vi "GetPrinterSettings.vi"(8 "error in (no error)":errorcluster, 11 "PrintDialog Refnum":refnum<k24>) -> (0 "error out":errorcluster, 2 "printer settings":T1, 3 "Refnum Out":refnum<k24>)   [LabVIEW 2015]
uses:
  System.Windows.Forms
  System.Drawing
panel:
  in  "margins (1.00)":T2={"top"=1.0, "left"=1.0, "right"=1.0, "bottom"=1.0} {"right" format="%.2f"; "bottom" format="%.2f"; "top" format="%.2f"; "left" format="%.2f"}
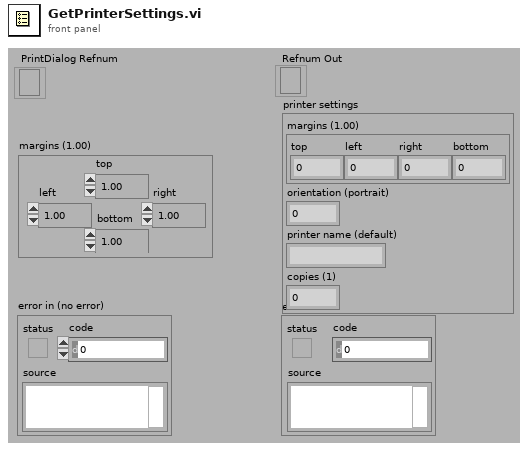
[diagram p1: front panel]
types:
  T1 = cluster{"margins (1.00)":cluster{"top":dbl, "left":dbl, "right":dbl, "bottom":dbl}, "orientation (portrait)":i32, "printer name (default)":string, "copies (1)":i16}
  T2 = cluster{"top":dbl, "left":dbl, "right":dbl, "bottom":dbl}
  T3 = cluster{"margins (1.00)":cluster{"top":dbl, "left":dbl, "right":dbl, "bottom":dbl}, "orientation (portrait)":i32, "PrinterName":string, "Copies":i16}
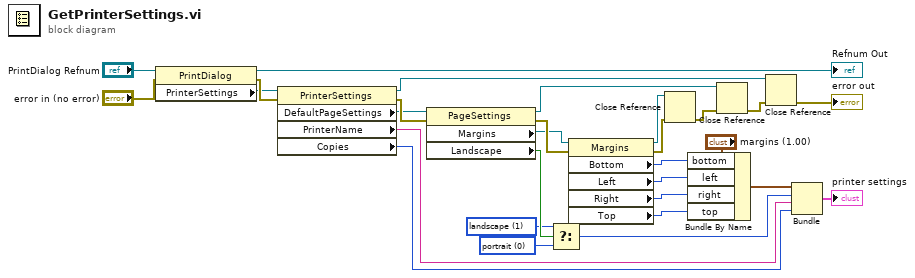
[diagram p0: block diagram]
diagram:
  w14 = 0 items=["portrait", "landscape"] ("orientation (portrait)")
  w15 = 1 items=["portrait", "landscape"] ("orientation (portrait)")
  n1 = property class="PrintDialog"(reference="PrintDialog Refnum", error in="error in (no error)") -> (reference out=→"Refnum Out":refnum<k24>, error out=w28:errorcluster, "PrinterSettings"=w25:refnum<k24>)
  n2 = property class="PrinterSettings"(reference=w25, error in=w28) -> (reference out=w9:refnum<k24>, error out=w29:errorcluster, "DefaultPageSettings"=w24:refnum<k24>, "PrinterName"=w3:string, "Copies"=w2:i16)
  n3 = property class="PageSettings"(reference=w24, error in=w29) -> (reference out=w8:refnum<k24>, error out=w23:errorcluster, "Margins"=w22:refnum<k24>, "Landscape"=w21:bool)
  n4 = Select(t=w15, s=w21, f=w14) -> (s? t:f=w4:i32)
  n5 = property class="Margins"(reference=w22, error in=w23) -> (reference out=w12:refnum<k24>, error out=w13:errorcluster, "Bottom"=w19:i32, "Left"=w18:i32, "Right"=w17:i32, "Top"=w16:i32)
  n6 = Close Reference(reference=w12, error in (no error)=w13) -> (error out=w11:errorcluster)
  n7 = Bundle By Name(cluster="margins (1.00)", "bottom"=w19, "left"=w18, "right"=w17, "top"=w16) -> (w5:T2)
  n8 = Close Reference(reference=w8, error in (no error)=w11) -> (error out=w10:errorcluster)
  n9 = Close Reference(reference=w9, error in (no error)=w10) -> (error out=→"error out":errorcluster)
  n10 = Bundle("margins (1.00)"=w5, "orientation (portrait)"=w4, "PrinterName"=w3, "Copies"=w2) -> (→"printer settings":T3)  [unwired: 1 out]
